vi "playFinishSound.vi"(8 "manual stop":bool, 11 "sounds":T1={"welcome sound"=path "C:/Users/wingX/Documents/WingXSVN/labview/daq test/sounds/welcome.wav", "play welcome"=TRUE, "got fly sound"=path "C:/Users/wingX/Documents/WingXSVN/labview/daq test/sounds/gotafly.wav", "play got fly"=FALSE, "discard sound"=path "C:/Users/wingX/Documents/WingXSVN/labview/daq test/sounds/blowingback.wav", "play discard"=FALSE, "finish sound"=path "C:/Users/wingX/Documents/WingXSVN/labview/daq test/sounds/finishedmeasuring.wav", "play finish"=TRUE, "inactivity alarm sound"=path "C:/Users/wingX/Documents/WingXSVN/labview/daq test/sounds/finishedmeasuring.wav", "play inactivity\nalarm"=TRUE}) -> ()   [LabVIEW 2012]
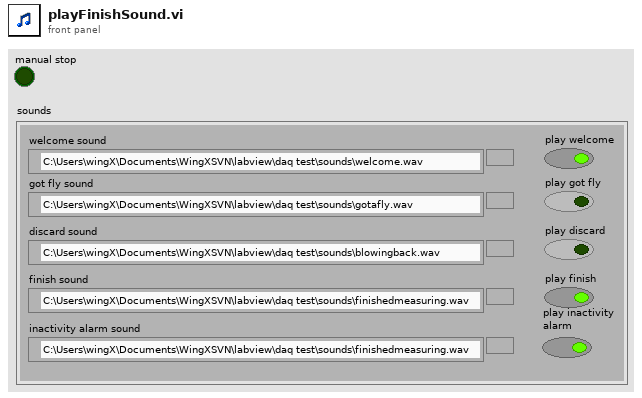
[diagram p1: front panel]
types:
  T1 = cluster{"welcome sound":path, "play welcome":bool, "got fly sound":path, "play got fly":bool, "discard sound":path, "play discard":bool, "finish sound":path, "play finish":bool, "inactivity alarm sound":path, "play inactivity\nalarm":bool}
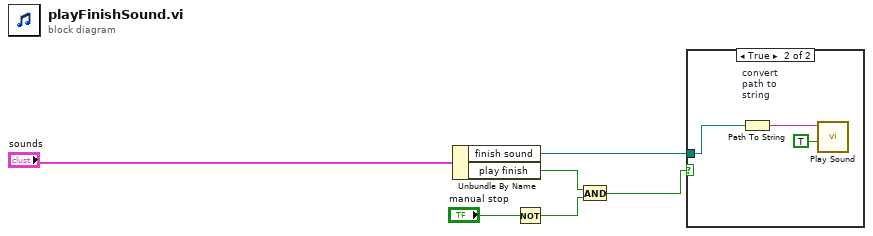
[diagram p0: block diagram]
diagram:
  n1 = Unbundle By Name("sounds") -> ("finish sound"=w6:path, "play finish"=w5:bool)
  n2 = Not(x="manual stop") -> (.not. x?=w3:bool)
  n3 = And(x=w5, y=w3) -> (x .and. y?=w4:bool)
  n4 = case shown="True" w4 {
    tunnel: w6 -> [_ w8]
    frame False {
    }
    frame True {
      n5 = Path To String "convert\npath to\nstring"(path=w8) -> (string=w9:string)
      n6 = call "Play Sound.vi"("Asynchronous? (F)"=TRUE, "Sound Name"=w9) -> ()  [unwired: 3 in, 1 out]
    }
  }
